vi "VT4002_Control.vi"() -> ()   [LabVIEW 2019]
uses:
  <userlib>/_TI-LA/Instr Drivers/Temperature Controller/Votsch4002/Driver/EasyIO/Typedefs/Instrument Model.ctl
  <userlib>/_TI-LA/Instr Drivers/Temperature Controller/Votsch4002/Driver/EasyIO/Typedefs/Votsch4002 Set Point Configuration.ctl
  <userlib>/_TI-LA/Instr Drivers/Temperature Controller/Votsch4002/Driver/Votsch4002.lvlib
panel:
  out "dup VISA resource name":refnum<visa-resource-name>
  out "error out":errorcluster
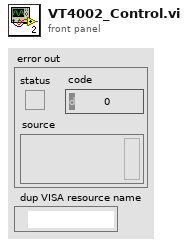
[diagram p1: front panel]
types:
  T1 = typedef "Votsch4002.lvlib/Votsch4002 Set Point Configuration.ctl" = cluster{"Address":string, "Temperature SetPoint":dbl}
  T2 = typedef "Votsch4002.lvlib/Instrument Model.ctl" = enum16{"Votsch 4002", "Votsch 4004", "Votsch 7004"}
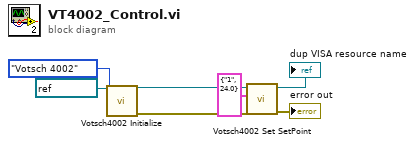
[diagram p0: block diagram]
diagram:
  n1 = call <userlib>:"Votsch4002 Initialize.vi"("VISA resource name"=refnum<visa-resource-name> "COM9", "Instrument Model"=Instrument_Model."Votsch 4002") -> ("VISA resource name out"=w5:refnum<visa-resource-name>, "error out"=w4:errorcluster)  [unwired: 12 in]
  n2 = call <userlib>:"Votsch4002 Set SetPoint.vi"("error in (no error)"=w4, "VT4002_Set Point"=T1 {"Address"="1", "Temperature SetPoint"=24.0}, "VISA resource name"=w5) -> ("error out"=→"error out":errorcluster, "dup VISA resource name"=→"dup VISA resource name":refnum<visa-resource-name>)  [unwired: 7 in]
